vi "IMUprocess.vi"(9 "Frames Read":u16[](array[numeric]), 11 "error in (no error)":errorcluster) -> (0 "error out":errorcluster, 2 "Gyro deg/s":dbl[](array[numeric]), 3 "Accel g's":dbl[](array[numeric]))   [LabVIEW 2016]
doc: "Inputs\nRaw data from MPU9250\n\nOutputs\nAccelerometer readings\nGyroscope redaings\n\nBitshifts the rawdata and put them in two arrays, one for accelerometer data and for gyroscope data"
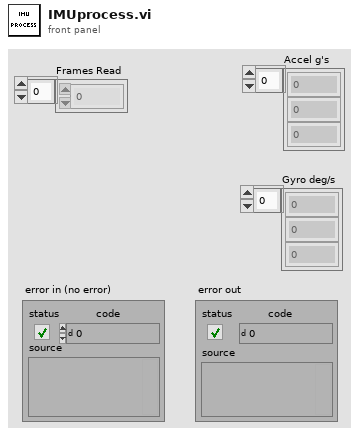
[diagram p1: front panel]
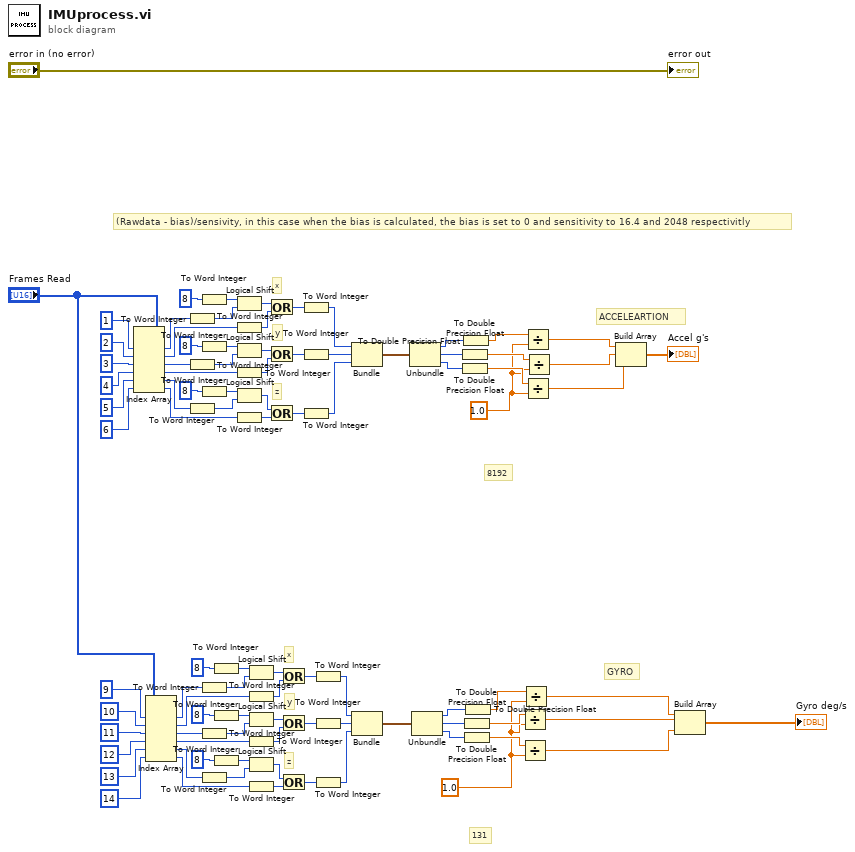
[diagram p0: block diagram]
diagram:
  w4 = 1.0
  w8 = 1.0
  # "131"
  # "8192"
  # "GYRO"
  # "(Rawdata - bias)/sensivity, in this case when the bias is calculated, the bias is set to 0 and sensitivity to 16.4 and 2048 respectivitly"
  # "ACCELEARTION"
  # "z"
  # "y"
  # "x"
  # "z"
  # "y"
  # "x"
  n1 = Index Array(array="Frames Read", index #1=1 ("index"), index #2=2 ("index"), index #3=3 ("index"), index #4=4 ("index"), index #5=5 ("index"), index #6=6 ("index")) -> (element #1=w40:u16, element #2=w45:u16, element #3=w53:u16, element #4=w57:u16, element #5=w62:u16, element #6=w63:u16)
  n2 = Index Array(array="Frames Read", index #1=9 ("index"), index #2=10 ("index"), index #3=11 ("index"), index #4=12 ("index"), index #5=13 ("index"), index #6=14 ("index")) -> (element #1=w83:u16, element #2=w84:u16, element #3=w85:u16, element #4=w86:u16, element #5=w87:u16, element #6=w88:u16)
  n3 = To Word Integer(number=w40) -> (16bit integer=w41:i16)
  n4 = To Word Integer(number=w53) -> (16bit integer=w56:i16)
  n5 = To Word Integer(number=w62) -> (16bit integer=w61:i16)
  n6 = To Word Integer(number=i16 8 ("y")) -> (16bit integer=w42:i16)
  n7 = To Word Integer(number=i16 8 ("y")) -> (16bit integer=w55:i16)
  n8 = To Word Integer(number=i16 8 ("y")) -> (16bit integer=w60:i16)
  n9 = To Word Integer(number=w83) -> (16bit integer=w76:i16)
  n10 = To Word Integer(number=w85) -> (16bit integer=w70:i16)
  n11 = To Word Integer(number=w87) -> (16bit integer=w66:i16)
  n12 = To Word Integer(number=i16 8 ("y")) -> (16bit integer=w75:i16)
  n13 = To Word Integer(number=i16 8 ("y")) -> (16bit integer=w71:i16)
  n14 = To Word Integer(number=i16 8 ("y")) -> (16bit integer=w67:i16)
  n15 = Logical Shift(y=w42, x=w41) -> (x << y=w23:i16)
  n16 = To Word Integer(number=w45) -> (16bit integer=w44:i16)
  n17 = Logical Shift(y=w55, x=w56) -> (x << y=w24:i16)
  n18 = To Word Integer(number=w57) -> (16bit integer=w58:i16)
  n19 = Logical Shift(y=w60, x=w61) -> (x << y=w25:i16)
  n20 = To Word Integer(number=w63) -> (16bit integer=w64:i16)
  n21 = Logical Shift(y=w75, x=w76) -> (x << y=w82:i16)
  n22 = To Word Integer(number=w84) -> (16bit integer=w73:i16)
  n23 = Logical Shift(y=w71, x=w70) -> (x << y=w81:i16)
  n24 = To Word Integer(number=w86) -> (16bit integer=w69:i16)
  n25 = Logical Shift(y=w67, x=w66) -> (x << y=w80:i16)
  n26 = To Word Integer(number=w88) -> (16bit integer=w65:i16)
  n27 = Or(x=w23, y=w44) -> (x .or. y?=w34:i16)
  n28 = Or(x=w24, y=w58) -> (x .or. y?=w38:i16)
  n29 = Or(x=w25, y=w64) -> (x .or. y?=w37:i16)
  n30 = Or(x=w82, y=w73) -> (x .or. y?=w79:i16)
  n31 = Or(x=w81, y=w69) -> (x .or. y?=w77:i16)
  n32 = Or(x=w80, y=w65) -> (x .or. y?=w78:i16)
  n33 = To Word Integer(number=w34) -> (16bit integer=w35:i16)
  n34 = To Word Integer(number=w38) -> (16bit integer=w36:i16)
  n35 = To Word Integer(number=w37) -> (16bit integer=w39:i16)
  n36 = To Word Integer(number=w79) -> (16bit integer=w89:i16)
  n37 = To Word Integer(number=w77) -> (16bit integer=w90:i16)
  n38 = To Word Integer(number=w78) -> (16bit integer=w91:i16)
  n39 = Bundle(w35, w36, w39) -> (w33:cluster{i16, i16, i16})  [unwired: 1 in]
  n40 = Bundle(w89, w90, w91) -> (w52:cluster{i16, i16, i16})  [unwired: 1 in]
  n41 = Unbundle(w33) -> (w46:i16, w47:i16, w48:i16)
  n42 = Unbundle(w52) -> (w51:i16, w50:i16, w49:i16)
  n43 = To Double Precision Float(number=w47) -> (double precision float=w13:dbl)
  n44 = To Double Precision Float(number=w48) -> (double precision float=w12:dbl)
  n45 = To Double Precision Float(number=w46) -> (double precision float=w14:dbl)
  n46 = To Double Precision Float(number=w50) -> (double precision float=w6:dbl)
  n47 = To Double Precision Float(number=w49) -> (double precision float=w5:dbl)
  n48 = To Double Precision Float(number=w51) -> (double precision float=w7:dbl)
  n49 = Divide(x=w6, y=w4) -> (x/y=w2:dbl)
  n50 = Divide(x=w5, y=w4) -> (x/y=w3:dbl)
  n51 = Divide(x=w7, y=w4) -> (x/y=w1:dbl)
  n52 = Divide(x=w14, y=w8) -> (x/y=w11:dbl)
  n53 = Divide(x=w12, y=w8) -> (x/y=w9:dbl)
  n54 = Divide(x=w13, y=w8) -> (x/y=w10:dbl)
  n55 = Build Array(w11, w10, w9) -> (→"Accel g's":dbl[])
  n56 = Build Array(w1, w2, w3) -> (→"Gyro deg/s":dbl[])
  "error out" <- "error in (no error)"
